vi "lsl get desc.vi"(8 "error in (no error)":errorcluster, 11 "streaminfo":T2) -> (0 "error out":errorcluster, 3 "xml_ptr":T1)   [LabVIEW 2018, in "liblsl-LabVIEW.lvlib"]
doc: "extern LIBLSL_C_API lsl_xml_ptr lsl_get_desc(lsl_streaminfo info);"
uses:
  <userlib>/liblsl-LabVIEW/liblsl-LabVIEW.lvlib
  <userlib>/liblsl-LabVIEW/Custom Controls/lsl_streaminfo.ctl
  <userlib>/liblsl-LabVIEW/Custom Controls/lsl_xml_ptr.ctl
  <userlib>/liblsl-LabVIEW/liblsl64.dll
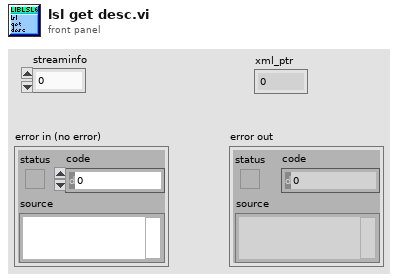
[diagram p1: front panel]
types:
  T1 = typedef "liblsl-LabVIEW.lvlib/lsl_xml_ptr.ctl" = u64
  T2 = typedef "liblsl-LabVIEW.lvlib/lsl_streaminfo.ctl" = u64
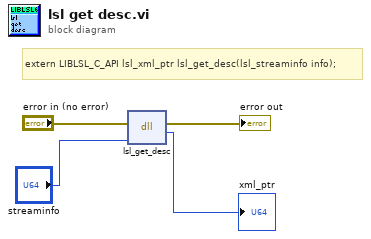
[diagram p0: block diagram]
diagram:
  # "extern LIBLSL_C_API lsl_xml_ptr lsl_get_desc(lsl_streaminfo info);"
  n1 = dll-call lib="C:/Program Files/National Instruments/LabVIEW 2018/user.lib/liblsl-LabVIEW/liblsl64.dll" fn="lsl_get_desc"(error in="error in (no error)", "info"="streaminfo") -> (error out=→"error out":errorcluster, "return type"=→"xml_ptr":u64)  [unwired: 3 in, 1 out]
